vi "RSNRPZ Get Range.vi"(8 "error in (no error)":errorcluster, 10 "Channel (1)":i32=1, 11 "VISA session":refnum<visa-resource-name> caption="VISA resource name") -> (0 "error out":errorcluster, 2 "Range":i32, 3 "dup VISA session":refnum<visa-resource-name> caption="VISA resource name")   [LabVIEW 2010]
doc: "This VI returns a measurement range in which the corresponding sensor is to perform a measurement.\n\nNote:\n\n1) This VI is not available for NRP-Z51\n\nRemote-control command(s):\nSENS:RANG?"
uses:
  rsnrpz_32.dll
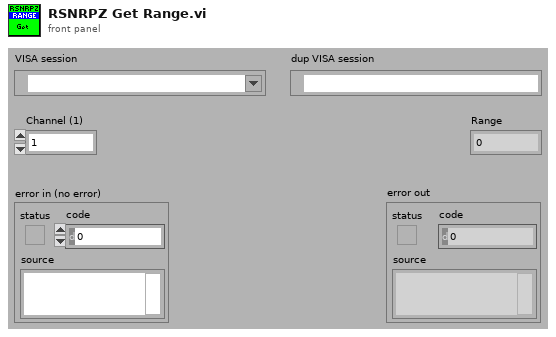
[diagram p1: front panel]
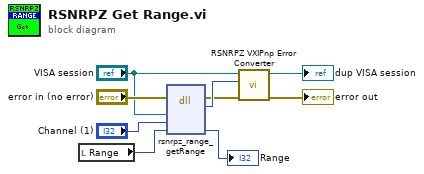
[diagram p0: block diagram]
diagram:
  n1 = local read "Range"() -> (w7:i32)
  n2 = dll-call lib="rsnrpz_32.dll" fn="rsnrpz_range_getRange"(error in="error in (no error)", "VISA Session"="VISA session", "Channel"="Channel (1)", "Range"=w7) -> (error out=w5:errorcluster, "Status"=w9:i32, "Range"=→"Range":i32)  [unwired: 4 in, 1 out]
  n3 = call <instrlib>:"RSNRPZ VXIPnp Error Converter.vi"("error in"=w5, "VXIPnp error code"=w9, "VISA session"="VISA session") -> ("error out"=→"error out":errorcluster, "dup VISA session"=→"dup VISA session":refnum<visa-resource-name>)  [unwired: 7 in]
